vi "Translate_Standard.vi"(6 "timeout (ms)(10000)":i32=10000, 7 "DeepL authKey":string, 8 "error in (no error)":errorcluster caption="エラー入力 (エラーなし)", 10 "TargetLang":T2, 11 "Input text":string) -> (0 "error out":errorcluster caption="エラー出力", 3 "translations":T1(array[cluster]))   [LabVIEW 2015, in "lv-deepl-api.lvlib"]
uses:
  lv-deepl-api.lvlib
  TargetLang.ctl
  <vilib>/httpClient/POSTBuffer.vi
  <vilib>/httpClient/LabVIEWHTTPClient.lvlib
panel:
  out "headers":string
  out "body":string
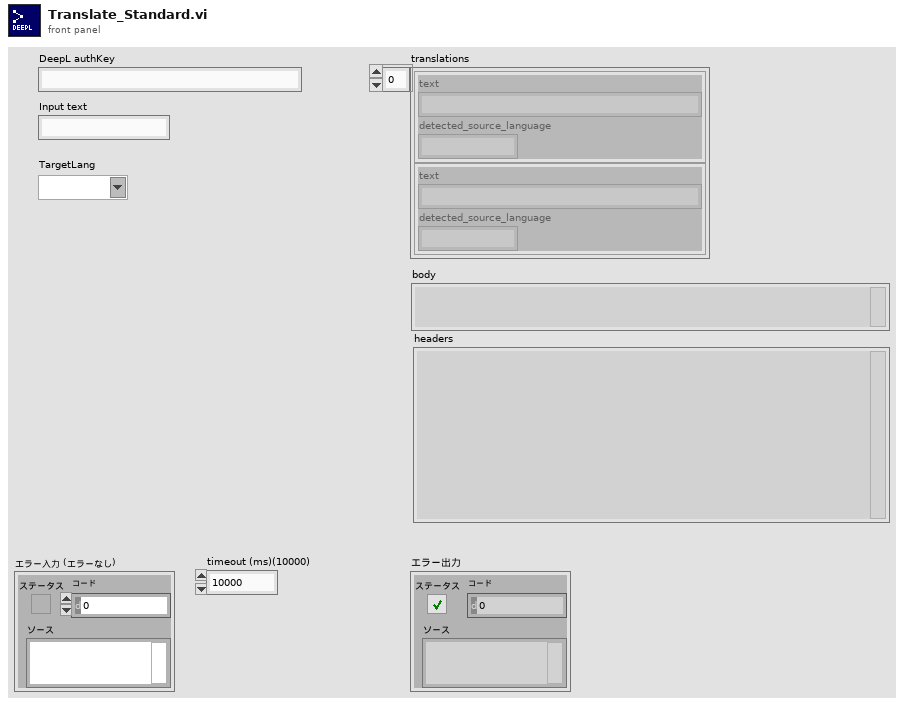
[diagram p1: front panel]
types:
  T1 = cluster{"detected_source_language":string, "text":string}[]
  T2 = typedef "lv-deepl-api.lvlib/TargetLang.ctl" = string
  T3 = typedef "LabVIEWHTTPClient.lvlib/ClientHandle.ctl" = refnum<k1>
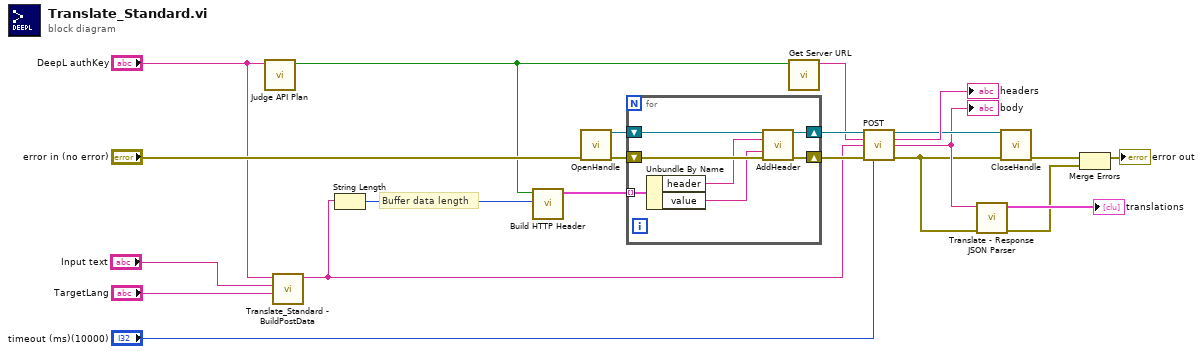
[diagram p0: block diagram]
diagram:
  # "Buffer data length"
  n1 = call "Judge API Plan.vi"("DeepL authKey"="DeepL authKey") -> ("DeepL Free API?"=w1:bool)  [unwired: 10 in]
  n2 = call "Translate_Standard - BuildPostData.vi"("TargetLang"="TargetLang", "Input text"="Input text", "DeepL authKey"="DeepL authKey") -> ("Post data"=w15:string)  [unwired: 8 in]
  n3 = String Length(string=w15) -> (length=w2:i32)
  n4 = call "Build HTTP Header.vi"("Numeric"=w2, "DeepL Free API?"=w1) -> ("Array"=w16:cluster{"header":string, "value":string}[])  [unwired: 9 in]
  n5 = call <vilib>:"OpenHandle.vi"("error in (no error)"="error in (no error)") -> ("client handle out"=w22:T3, "error out"=w21:errorcluster)  [unwired: 13 in]
  n6 = for {
    shift-right: [w27] -> w20
    shift-left: w22 -> [w29]
    shift-right: [w26] -> w19
    shift-left: w21 -> [w28]
    tunnel: w16 -> [w25] mode=indexing
    n7 = Unbundle By Name(w25) -> ("header"=w24:string, "value"=w23:string)
    n8 = call <vilib>:"AddHeader.vi"("client handle"=w29, "header"=w24, "value"=w23, "error in (no error)"=w28) -> ("client handle out"=w27:T3, "error out"=w26:errorcluster)  [unwired: 10 in]
  }
  n9 = call "Get Server URL.vi"("DeepL Free API?"=w1) -> ("url"=w5:string)  [unwired: 10 in]
  n10 = call-poly <vilib>:"POST.vi"("client handle"=w20, "url"=w5, "buffer"=w15, "error in (no error)"=w19, "timeout (10000)"="timeout (ms)(10000)") -> ("client handle out"=w17:T3, "headers"=→"headers":string, "body"=w12:string, "error out"=w4:errorcluster)  [unwired: 7 in]
  "body" <- w12
  n11 = call "Translate - Response JSON Parser.vi"("error in (no error)"=w4, "JSON Text"=w12) -> ("error out"=w9:errorcluster, "translations"=→"translations":T1)  [unwired: 8 in]
  n12 = call <vilib>:"CloseHandle.vi"("client handle"=w17, "error in (no error)"=w4) -> ("error out"=w10:errorcluster)  [unwired: 13 in]
  n13 = Merge Errors(w10, w9) -> (→"error out":errorcluster)
